vi "programacion puntos extras.vi"() -> ()   [LabVIEW 2011]
panel:
  out "Array":dbl[](array[numeric])
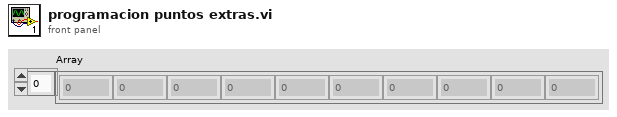
[diagram p1: front panel]
types:
  T1 = enum16{"open", "replace", "create", "open or create", "replace or create", "replace or create with confirmation"}
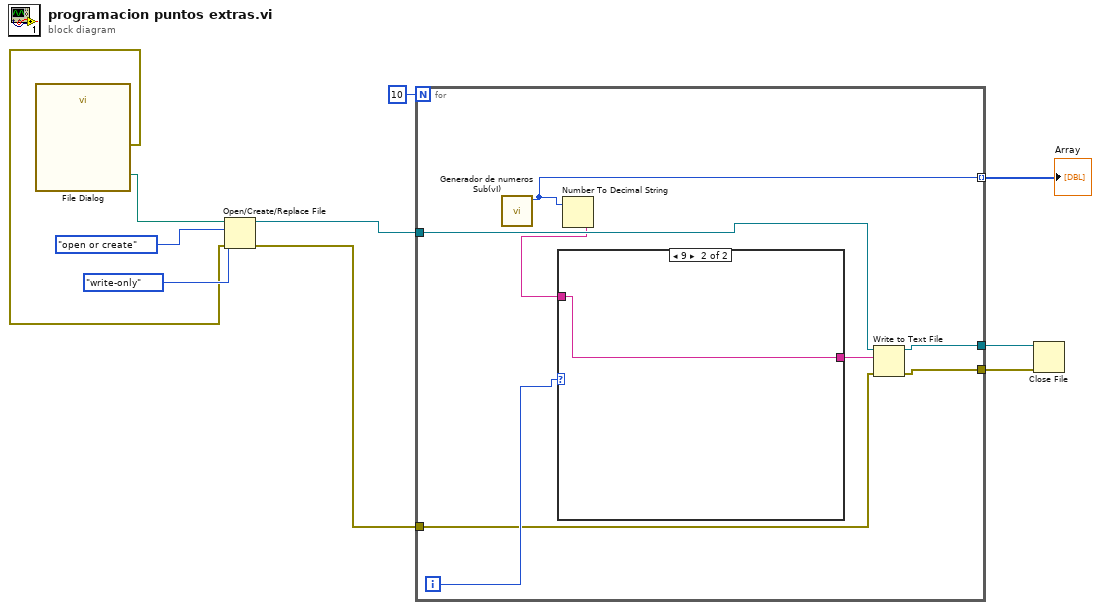
[diagram p0: block diagram]
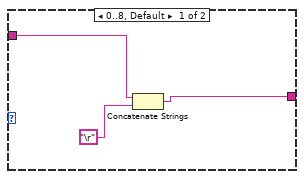
[diagram p2: hidden frame]
diagram:
  n1 = call "File Dialog"() -> ("selected path"=w10:path, "error out"=w7:errorcluster)  [unwired: 12 in, 2 out]
  n2 = Open/Create/Replace File(file path (use dialog)=w10, error in=w7, operation (0:open)=T1."open or create", access (0:read/write)=enum16{"read/write", "read-only", "write-only"}."write-only") -> (refnum out=w4:refnum<file>, error out=w3:errorcluster)  [unwired: 2 in, 1 out]
  n3 = for {
    N: 10 -> [_]
    tunnel: [w15] -> w5 mode=indexing
    tunnel: w4 -> [w17]
    tunnel: w3 -> [w16]
    tunnel: [w12] -> w2
    tunnel: [w11] -> w1
    i -> [w18]
    n4 = call "Generador de numeros Sub(vI).vi"() -> ("Numeric"=w15:i32)  [unwired: 11 in]
    n5 = Number To Decimal String(number=w15) -> (decimal integer string=w14:string)  [unwired: 1 in]
    n6 = case shown="9" w18 {
      tunnel: w14 -> [w21 w22]
      tunnel: [w19 w22] -> w13
      frame 0..8, Default {
        n7 = Concatenate Strings(w21, "\r") -> (w19:string)
      }
      frame 9 {
      }
    }
    n8 = Write to Text File(file (use dialog)=w17, text=w13, error in=w16) -> (refnum out=w12:refnum<file>, error out=w11:errorcluster)  [unwired: 1 in, 1 out]
  }
  "Array" <- w5
  n9 = Close File(refnum=w2, error in=w1) -> ()  [unwired: 2 out]
